vi "报警方式处理模块-网络版.vi"(5 "串口配置":T1, 7 "连接ID":refnum<k5>, 9 "硬件限值":dbl caption="限值1", 10 "硬件未报警？":bool, 11 "报警方式 i":T2) -> (2 "值改变？":bool, 3 "报警方式 o":T2)   [LabVIEW 2017]
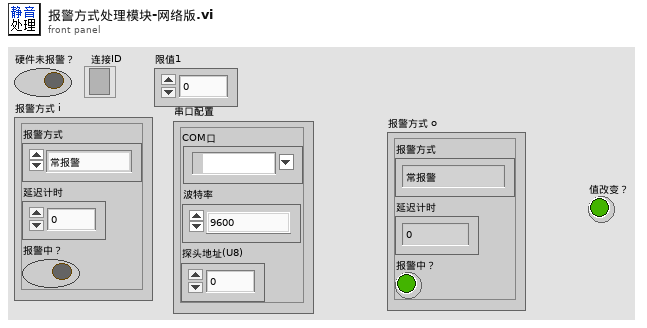
[diagram p1: front panel]
types:
  T1 = typedef "串口配置.ctl" = cluster{"COM口":refnum<visa-resource-name>, "波特率":enum16{"9600", "19200"}, "探头地址(U8)":u8}
  T2 = cluster{"报警方式":enum16{"常报警", "自动静音", "手动静音"}, "延迟计时":u16, "报警中？":bool}
  T3 = typedef "串口模块输入.ctl" = cluster{"串口动作类型":T4, "串口配置":T1, "数据输入":variant}
  T4 = typedef "串口动作类型.ctl" = enum16{"读测量值", "设置报警值", "设置地址", "设置系数", "广播修改波特率", "关闭串口"}
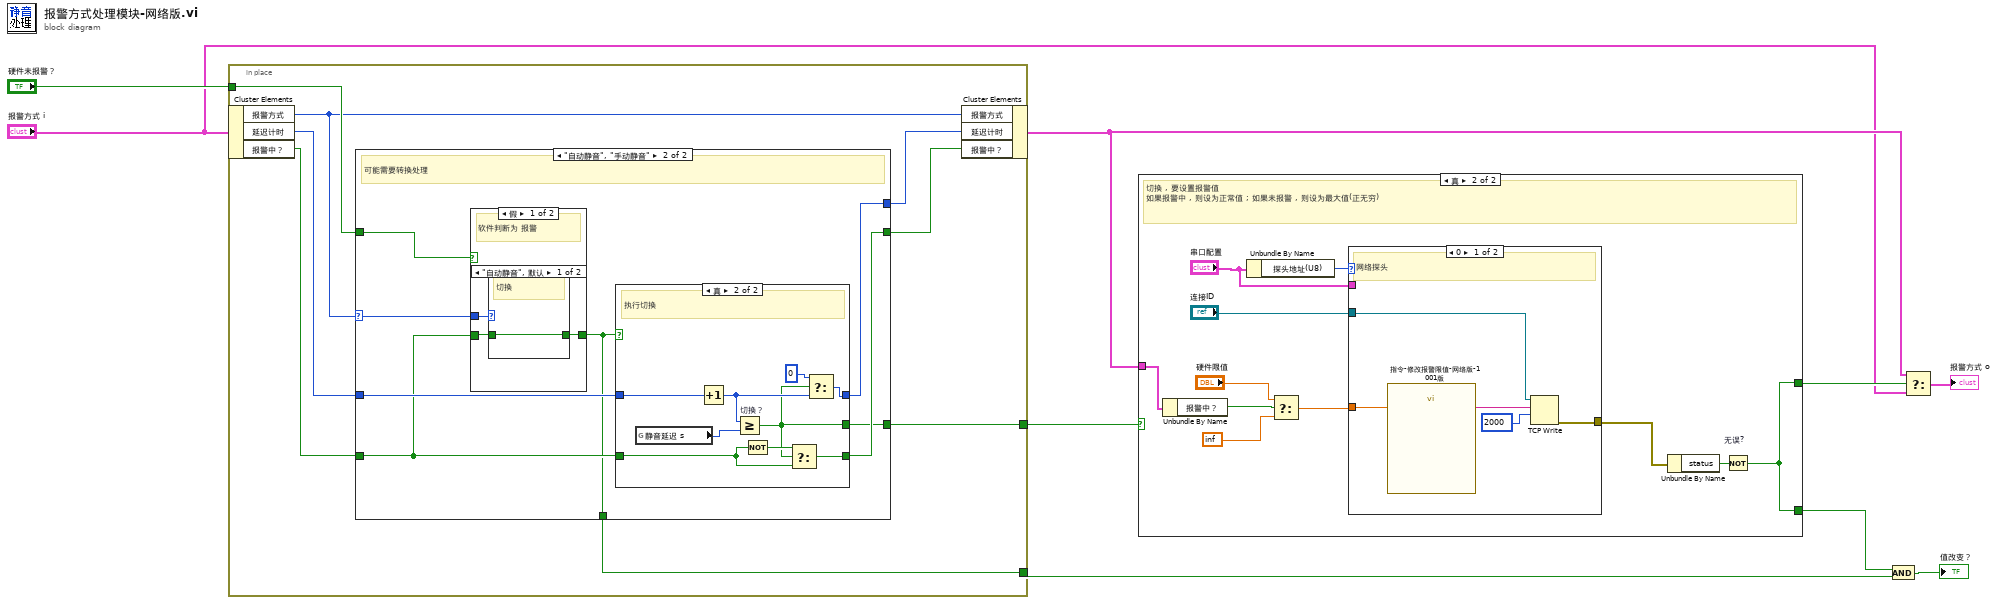
[diagram p0: block diagram]
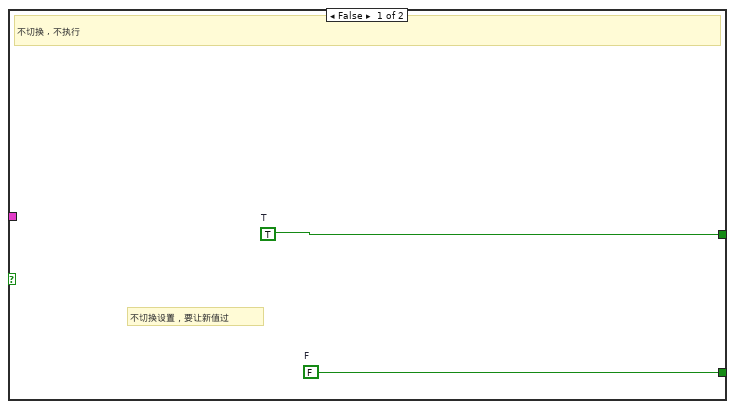
[diagram p2: hidden frame]
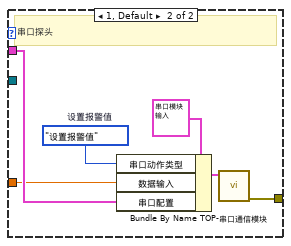
[diagram p3: hidden frame]
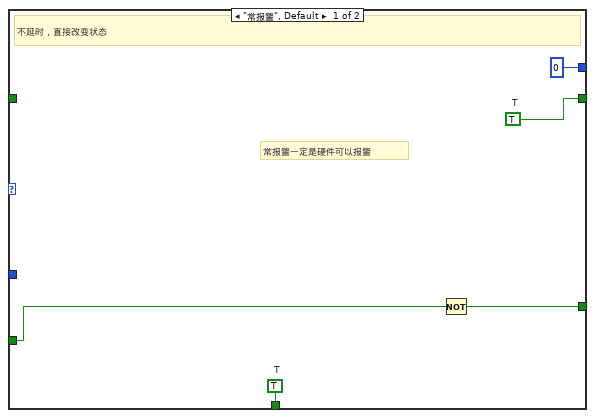
[diagram p4: hidden frame]
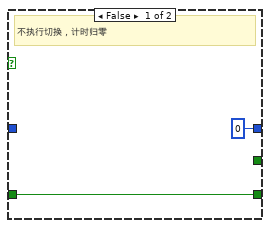
[diagram p5: hidden frame]
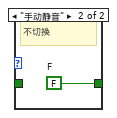
[diagram p6: hidden frame]
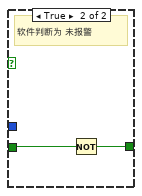
[diagram p7: hidden frame]
diagram:
  n1 = in-place {
    in-place-border: "硬件未报警？" -> [w17]
    in-place-border: [w12] -> w8
    in-place-border: [w10] -> w1
    n2 = in-place-cluster #1("报警方式 i") -> ("报警方式"=w13:enum16{"常报警", "自动静音", "手动静音"}, "延迟计时"=w14:u16, "报警中？"=w16:bool)
    n3 = case shown="\"自动静音\", \"手动静音\"" w13 {
      selector: w13 -> [_ w29]
      tunnel: w17 -> [_ w30]
      tunnel: w16 -> [w19 w26]
      tunnel: [0 w27] -> w15
      tunnel: [w20 w25] -> w11
      tunnel: w14 -> [_ w28]
      tunnel: [w18 w24] -> w12
      tunnel: [w21 w23] -> w10
      frame "常报警", Default {
        w20 = TRUE  # T
        w21 = TRUE  # T
        # "常报警一定是硬件可以报警"
        # "不延时，直接改变状态"
        n4 = Not(x=w19) -> (.not. x?=w18:bool)
      }
      frame "自动静音", "手动静音" {
        # "可能需要转换处理"
        n5 = case shown="假" w30 {
          tunnel: w26 -> [w42 w48]
          tunnel: [w43 w47] -> w23
          tunnel: w29 -> [w44 _]
          frame False {
            # "软件判断为 报警"
            n6 = case shown="\"自动静音\", 默认" w44 {
              tunnel: [w45 w46] -> w43
              tunnel: w42 -> [w45 _]
              frame "自动静音", Default {
                # "切换"
              }
              frame "手动静音" {
                w46 = FALSE  # F
                # "不切换"
              }
            }
          }
          frame True {
            # "软件判断为 未报警"
            n7 = Not(x=w48) -> (.not. x?=w47:bool)
          }
        }
        n8 = case shown="真" w23 {
          tunnel: w28 -> [_ w40]
          tunnel: [0 w38] -> w27
          tunnel: w26 -> [w32 w37]
          tunnel: [w32 w35] -> w25
          tunnel: [_ w34] -> w24
          frame False {
            # "不执行切换，计时归零"
          }
          frame True {
            # "执行切换"
            n9 = global read "全局变量-35点监测.vi" "静音延迟 s"() -> (w33:u16)
            n10 = Increment(x=w40) -> (x+1=w39:u16)
            n11 = Greater Or Equal? "切换？"(x=w39, y=w33) -> (x >= y?=w34:bool)
            n12 = Not(x=w37) -> (.not. x?=w36:bool)
            n13 = Select(t=w36, s=w34, f=w37) -> (s? t:f=w35:bool)
            n14 = Select(t=0, s=w34, f=w39) -> (s? t:f=w38:i32)
          }
        }
      }
    }
    n15 = in-place-cluster #1("报警方式"=w13, "延迟计时"=w15, "报警中？"=w11) -> (w5:T2)
  }
  n16 = case shown="真" w8 {
    tunnel: w5 -> [_ w61]
    tunnel: [w50 w53] -> w6
    tunnel: [w49 w53] -> w2
    frame False {
      w49 = FALSE  # F
      w50 = TRUE  # T
      # "不切换设置，要让新值过"
      # "不切换 , 不执行"
    }
    frame True {
      # "切换 , 要设置报警值\n如果报警中 , 则设为正常值 ; 如果未报警 , 则设为最大值(正无穷)"
      n17 = Unbundle By Name(w61) -> ("报警中？"=w60:bool)
      n18 = Unbundle By Name("串口配置") -> ("探头地址(U8)"=w52:u8)
      n19 = Select(t="硬件限值", s=w60, f=inf) -> (s? t:f=w57:dbl)
      n20 = case shown="0" w52 {
        tunnel: w57 -> [w64 w68]
        tunnel: "连接ID" -> [w63 _]
        tunnel: [w62 w67] -> w55
        tunnel: "串口配置" -> [_ w69]
        frame 0 {
          # "网络探头"
          n21 = call "指令-修改报警限值-网络版-1001版.vi"("限值"=w64) -> ("指令输出"=w66:string)  [unwired: 10 in]
          n22 = TCP Write(connection ID=w63, data in=w66, 9:2000 ("超时毫秒(25000)")) -> (error out=w62:errorcluster)  [unwired: 1 in, 2 out]
        }
        frame 1, Default {
          w70 = 串口动作类型."设置报警值"  # 设置报警值
          # "串口探头"
          n23 = Bundle By Name(cluster=T3 {"串口动作类型"=enum."读测量值", "串口配置"={"COM口"="", "波特率"=enum."9600", "探头地址(U8)"=0}, "数据输入"=variant} ("串口模块输入"), "串口动作类型"=w70, "数据输入"=w68, "串口配置"=w69) -> (w72:T3)
          n24 = call "TOP-串口通信模块.vi"("串口模块输入"=w72) -> ("error out"=w67:errorcluster)  [unwired: 9 in, 1 out]
        }
      }
      n25 = Unbundle By Name(w55) -> ("status"=w54:bool)
      n26 = Not "无误?"(x=w54) -> (.not. x?=w53:bool)
    }
  }
  n27 = And(x=w2, y=w1) -> (x .and. y?=→"值改变？":bool)
  n28 = Select(t=w5, s=w6, f="报警方式 i") -> (s? t:f=→"报警方式 o":T2)
